vi "sequence.vi"() -> ()   [LabVIEW 2015]
panel:
  out "2":dbl
  out "1":dbl
  out "計時":dbl
  # "同時執行"
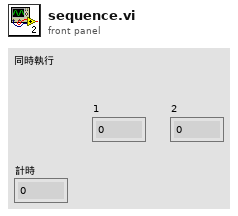
[diagram p1: front panel]
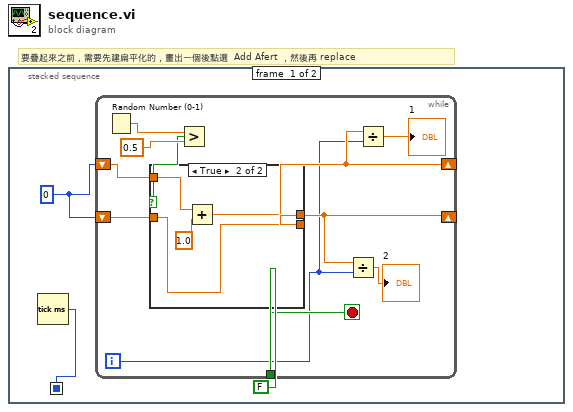
[diagram p0: block diagram]
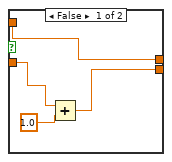
[diagram p2: hidden frame]
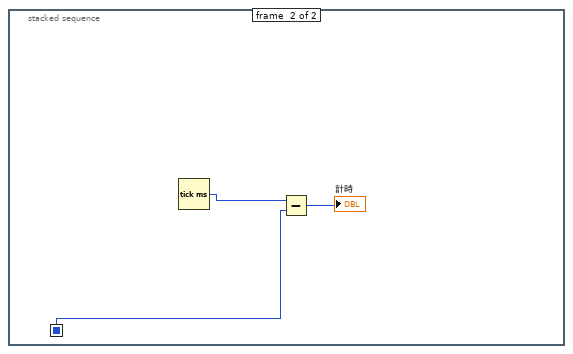
[diagram p3: hidden frame]
diagram:
  # "要疊起來之前，需要先建扁平化的，畫出一個後點選  Add Afert ，然後再 replace"
  n1 = stacked-sequence {
    seq-local: [w1 _] -> [_ w24]
    frame #0 {
      w3 = 0
      n2 = Tick Count (ms)() -> (millisecond timer value=w1:u32)
      n3 = while {
        shift-right: [w6] -> _
        shift-left: w3 -> [w11]
        shift-right: [w8] -> _
        shift-left: w3 -> [w10]
        tunnel: FALSE -> [w9]
        i -> [w4]
        stop <- w9 stop-if-true
        n4 = Random Number (0-1)() -> (number: 0 to 1=w13:dbl)
        n5 = Greater?(x=w13, y=0.5 ("x")) -> (0:w12:bool)
        n6 = case shown="True" w12 {
          tunnel: w11 -> [w15 w21]
          tunnel: [w15 w20] -> w6
          tunnel: w10 -> [w18 w19]
          tunnel: [w16 w19] -> w8
          frame False {
            n7 = Add(x=w18, y=1.0 ("x+y")) -> (x+y=w16:dbl)
          }
          frame True {
            n8 = Add(x=w21, y=1.0) -> (x+y=w20:dbl)
          }
        }
        n9 = Divide(x=w8, y=w4) -> (x/y=→"2":dbl)
        n10 = Divide(x=w6, y=w4) -> (x/y=→"1":dbl)
      }
    }
    frame #1 {
      n11 = Tick Count (ms)() -> (millisecond timer value=w25:u32)
      n12 = Subtract(x=w25, y=w24) -> (x-y=→"計時":u32)
    }
  }
